vi "Initialize.vi"(8 "error in (no error)":errorcluster, 10 "Device":string) -> (0 "error out":errorcluster, 3 "Oscilloscope":refnum<class "Oscilloscope.lvclass">)   [LabVIEW 2018, in "Oscilloscope.lvlib" / "Oscilloscope.lvclass"]
doc: "This method is used to get Configuration settings for the Oscope."
uses:
  Oscilloscope.lvclass
  Oscilloscope.lvclass/Oscilloscope.ctl
  PPLs/Configuration/Configuration.lvlibp/Configuration.lvclass
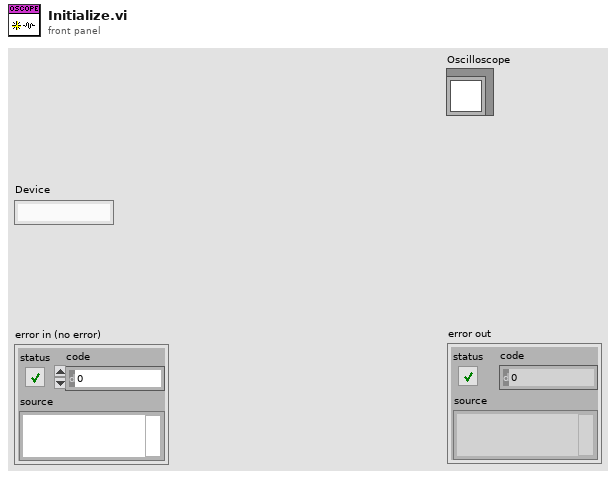
[diagram p1: front panel]
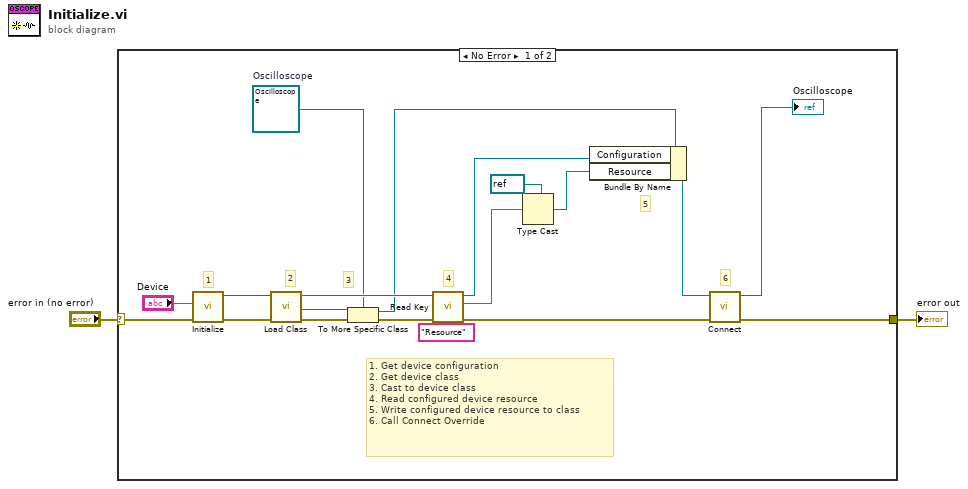
[diagram p0: block diagram]
diagram:
  n1 = case shown="No Error" "error in (no error)" {
    selector: "error in (no error)" -> [w20 w22]
    tunnel: [w5 w22] -> w1
    frame No Error {
      w7 = refnum<class "Oscilloscope.lvclass"> refnum  # Oscilloscope
      # "6"
      # "1. Get device configuration\n2. Get device class\n3. Cast to device class\n4. Read configured device resource\n5. Write configured device resource to class\n6. Call Connect Override"
      # "5"
      # "4"
      # "3"
      # "2"
      # "1"
      n2 = call "Initialize.vi"("error in"=w20, "Device"="Device") -> ("error out"=w19:errorcluster, "Configuration out"=w18:refnum<class "Configuration.lvclass">)  [unwired: 8 in]
      n3 = call "Load Class.vi"("error in"=w19, "Configuration in"=w18) -> ("error out"=w16:errorcluster, "Class out"=w17:refnum<class>, "Configuration out"=w14:refnum<class "Configuration.lvclass">)  [unwired: 7 in]
      n4 = To More Specific Class(target class=w7, reference=w17, error in=w16) -> (specific class reference=w13:refnum<class "Oscilloscope.lvclass">, error out=w15:errorcluster)
      n5 = call "Read Key.vi"("Key:"="Resource", "error in"=w15, "Configuration in"=w14) -> ("error out"=w6:errorcluster, "Value"=w10:string, "Configuration out"=w11:refnum<class "Configuration.lvclass">)  [unwired: 6 in]
      n6 = Type Cast(type=refnum<visa-resource-name> refnum ("VISA resource name"), x=w10) -> (*(type *) &x=w8:refnum<visa-resource-name>)
      n7 = Bundle By Name(cluster=w13, "Configuration"=w11, "Resource"=w8) -> (w4:refnum<class "Oscilloscope.lvclass">)
      n8 = call-dynamic "Connect.vi"("error in (no error)"=w6, "Oscilloscope in"=w4) -> ("error out"=w5:errorcluster, "Oscilloscope out"=→"Oscilloscope":refnum<class "Oscilloscope.lvclass">)  [unwired: 8 in]
    }
    frame Error {
    }
  }
  "error out" <- w1
